vi "test Loopback RT to BC with Start Stop and Status.vi"(8 "error in":errorcluster, 11 "TestCase in":refnum<class "Loopback.lvclass">) -> (0 "error out":errorcluster, 3 "TestCase out":refnum<class "Loopback.lvclass">)   [LabVIEW 2020, in "Loopback.lvclass"]
uses:
  Loopback.lvclass
  C:/dev/niveristand-custom-device-testing-tools/VeriStandTestCase/VeriStandTestCase.lvclass
  <vilib>/numeric/Random Number (Range) U64.vi
  485b7c2b-8320-4722-9ec7-d01f27c65546.vi
  1571aa8d-489e-4c94-925a-256c0ab49a50.vi
  a09b07c8-52ad-4e58-9957-78b331af32de.vi
  9426a44b-b3d4-42e7-bade-e6518c4f8208.vi
  <vilib>/numeric/sub_Random U32.vi
  <vilib>/NI VeriStand/Execution/Workspace/NI VeriStand - Set Multiple Channel Values.vi
  <vilib>/NI VeriStand/Execution/Workspace/NI VeriStand - Get Multiple Channel Values.vi
  <vilib>/NI VeriStand/Execution/Workspace/NI VeriStand - Set Single Channel Value.vi
  <vilib>/addons/_JKI Toolkits/VI Tester/TestCase.llb/TestCase.lvclass
  <vilib>/NI VeriStand/Execution/Workspace/NI_VS Workspace ExecutionAPI.lvlib
  C:/Program Files (x86)/National Instruments/LabVIEW 2020/vi.lib/addons/_JKI Toolkits/VI Tester/TestCase.llb/TestCase.lvclass
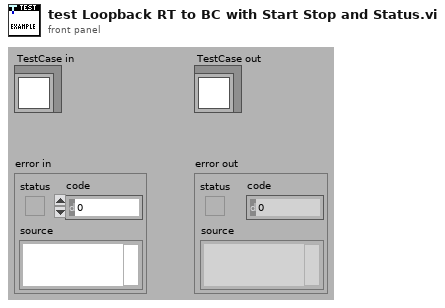
[diagram p1: front panel]
types:
  T1 = typedef "NI_VS Workspace ExecutionAPI.lvlib/WorkspaceAPI.ctl" = refnum<k24>
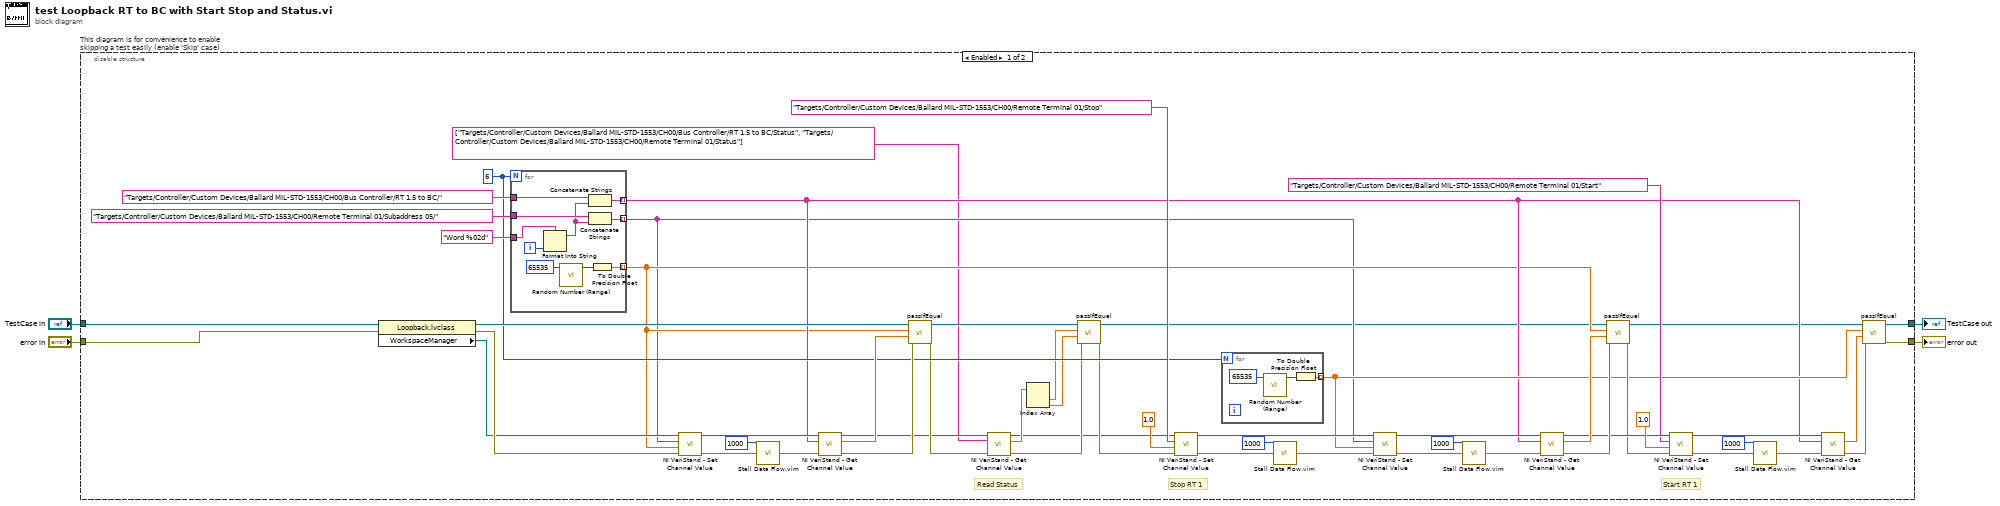
[diagram p0: block diagram]
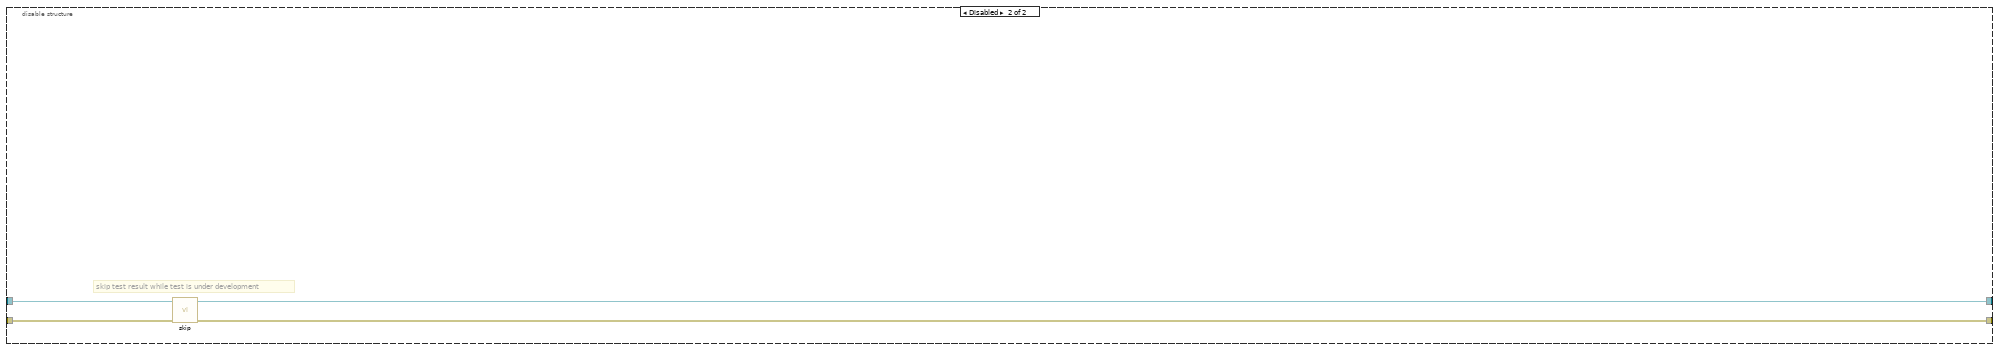
[diagram p2: hidden frame]
diagram:
  n1 = disable-structure "This diagram is for convenience to enable skipping a test easily (enable 'Skip' case)" shown="Enabled" {
    disable-tunnel: "TestCase in" -> [w50 w76]
    disable-tunnel: [w17 w74] -> w1
    disable-tunnel: [w19 w75] -> w3
    disable-tunnel: "error in" -> [w47 w73]
    frame Enabled {
      w22 = 6
      # "Read Status"
      # "Start RT 1"
      # "Stop RT 1"
      n2 = property class="Loopback.lvclass"(reference=w50, error in=w47) -> (reference out=w59:refnum<class "Loopback.lvclass">, error out=w54:errorcluster, "WorkspaceManager"=w52:T1)
      n3 = for {
        N: w22 -> [_]
        tunnel: "Targets/Controller/Custom Devices/Ballard MIL-STD-1553/CH00/Remote Terminal 01/Subaddress 05/" ("Channel") -> [w68]
        tunnel: [w69] -> w16 mode=indexing
        tunnel: "Targets/Controller/Custom Devices/Ballard MIL-STD-1553/CH00/Bus Controller/RT 1.5 to BC/" ("Channel") -> [w67]
        tunnel: [w66] -> w21 mode=indexing
        tunnel: "Word %02d" -> [w60]
        tunnel: [w61] -> w20 mode=indexing
        i -> [w65]
        n4 = Format Into String(format string=w60, w65) -> (resulting string=w64:string)  [unwired: 2 in, 1 out]
        n5 = call-poly <vilib>:"Random Number (Range).vi"("upper bound (100)"=u64 65535) -> ("number"=w63:u64)  [unwired: 10 in]
        n6 = Concatenate Strings(w67, w64) -> (w66:string)
        n7 = Concatenate Strings(w68, w64) -> (w69:string)
        n8 = To Double Precision Float(number=w63) -> (double precision float=w61:dbl)
      }
      n9 = call-poly <vilib>:"NI VeriStand - Set Channel Value.vi"("error in (no error)"=w54, "Values"=w20, "Channels"=w16, "WorkspaceManager in"=w52) -> ("error out"=w56:errorcluster, "WorkspaceManager out"=w58:T1)  [unwired: 6 in]
      n10 = call "Stall Data Flow.vim"("value in"=w56, "milliseconds to wait"=u32 1000) -> ("value out"=w57:errorcluster)  [unwired: 1 out]
      n11 = call-poly <vilib>:"NI VeriStand - Get Channel Value.vi"("error in (no error)"=w57, "Channels"=w21, "WorkspaceManager in"=w58) -> ("error out"=w53:errorcluster, "Values"=w51:dbl[], "WorkspaceManager out"=w8:T1)  [unwired: 6 in]
      n12 = call-dynamic "passIfEqual.vi"("error in (no error)"=w53, "y"=w51, "x"=w20, "TestCase in"=w59) -> ("error out"=w13:errorcluster, "TestCase out"=w12:refnum<class "Loopback.lvclass">)  [unwired: 6 in]
      n13 = call-poly <vilib>:"NI VeriStand - Get Channel Value.vi"("error in (no error)"=w13, "Channels"=string[] ["Targets/Controller/Custom Devices/Ballard MIL-STD-1553/CH00/Bus Controller/RT 1.5 to BC/Status", "Targets/Controller/Custom Devices/Ballard MIL-STD-1553/CH00/Remote Terminal 01/Status"], "WorkspaceManager in"=w8) -> ("error out"=w14:errorcluster, "Values"=w15:dbl[], "WorkspaceManager out"=w7:T1)  [unwired: 6 in]
      n14 = Index Array(array=w15) -> (element #1=w11:dbl, element #2=w10:dbl)  [unwired: 2 in]
      n15 = call-dynamic "passIfEqual.vi"("error in (no error)"=w14, "y"=w10, "x"=w11, "TestCase in"=w12) -> ("error out"=w9:errorcluster, "TestCase out"=w6:refnum<class "Loopback.lvclass">)  [unwired: 6 in]
      n16 = call-poly <vilib>:"NI VeriStand - Set Channel Value.vi"("error in (no error)"=w9, "Value"=1.0, "Channel"="Targets/Controller/Custom Devices/Ballard MIL-STD-1553/CH00/Remote Terminal 01/Stop", "WorkspaceManager in"=w7) -> ("error out"=w24:errorcluster, "WorkspaceManager out"=w43:T1)  [unwired: 6 in]
      n17 = for {
        N: w22 -> [_]
        tunnel: [w70] -> w29 mode=indexing
        n18 = call-poly <vilib>:"Random Number (Range).vi"("upper bound (100)"=u64 65535) -> ("number"=w71:u64)  [unwired: 10 in]
        n19 = To Double Precision Float(number=w71) -> (double precision float=w70:dbl)
      }
      n20 = call "Stall Data Flow.vim"("value in"=w24, "milliseconds to wait"=u32 1000) -> ("value out"=w23:errorcluster)  [unwired: 1 out]
      n21 = call-poly <vilib>:"NI VeriStand - Set Channel Value.vi"("error in (no error)"=w23, "Values"=w29, "Channels"=w16, "WorkspaceManager in"=w43) -> ("error out"=w27:errorcluster, "WorkspaceManager out"=w42:T1)  [unwired: 6 in]
      n22 = call "Stall Data Flow.vim"("value in"=w27, "milliseconds to wait"=u32 1000) -> ("value out"=w26:errorcluster)  [unwired: 1 out]
      n23 = call-poly <vilib>:"NI VeriStand - Get Channel Value.vi"("error in (no error)"=w26, "Channels"=w21, "WorkspaceManager in"=w42) -> ("error out"=w41:errorcluster, "Values"=w40:dbl[], "WorkspaceManager out"=w38:T1)  [unwired: 6 in]
      n24 = call-dynamic "passIfEqual.vi"("error in (no error)"=w41, "y"=w40, "x"=w20, "TestCase in"=w6) -> ("error out"=w34:errorcluster, "TestCase out"=w18:refnum<class "Loopback.lvclass">)  [unwired: 6 in]
      n25 = call-poly <vilib>:"NI VeriStand - Set Channel Value.vi"("error in (no error)"=w34, "Value"=1.0, "Channel"="Targets/Controller/Custom Devices/Ballard MIL-STD-1553/CH00/Remote Terminal 01/Start", "WorkspaceManager in"=w38) -> ("error out"=w35:errorcluster, "WorkspaceManager out"=w30:T1)  [unwired: 6 in]
      n26 = call "Stall Data Flow.vim"("value in"=w35, "milliseconds to wait"=u32 1000) -> ("value out"=w31:errorcluster)  [unwired: 1 out]
      n27 = call-poly <vilib>:"NI VeriStand - Get Channel Value.vi"("error in (no error)"=w31, "Channels"=w21, "WorkspaceManager in"=w30) -> ("error out"=w32:errorcluster, "Values"=w33:dbl[])  [unwired: 6 in, 1 out]
      n28 = call-dynamic "passIfEqual.vi"("error in (no error)"=w32, "y"=w33, "x"=w29, "TestCase in"=w18) -> ("error out"=w19:errorcluster, "TestCase out"=w17:refnum<class "Loopback.lvclass">)  [unwired: 6 in]
    }
    frame Disabled {
      # "skip test result while test is under development"
      n29 = call <vilib>:"skip.vi"("error in (no error)"=w73, "TestCase in"=w76) -> ("error out"=w75:errorcluster, "TestCase out"=w74:refnum<class "Loopback.lvclass">)  [unwired: 8 in]
    }
  }
  "error out" <- w3
  "TestCase out" <- w1
